vi "JKISM++ Example - Message API.vi"() -> ()   [LabVIEW 2014]
uses:
  user.lib/_NEVSTOP/JKI State Machine++/JKI State Machine++.lvlib
panel:
  out "Arguments 3":string
  out "Arguments 2":string
  out "Arguments":string
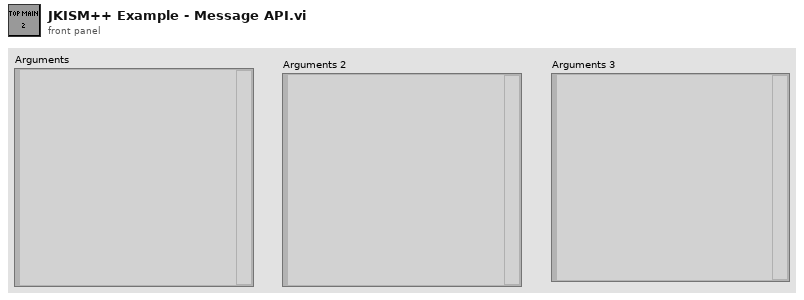
[diagram p1: front panel]
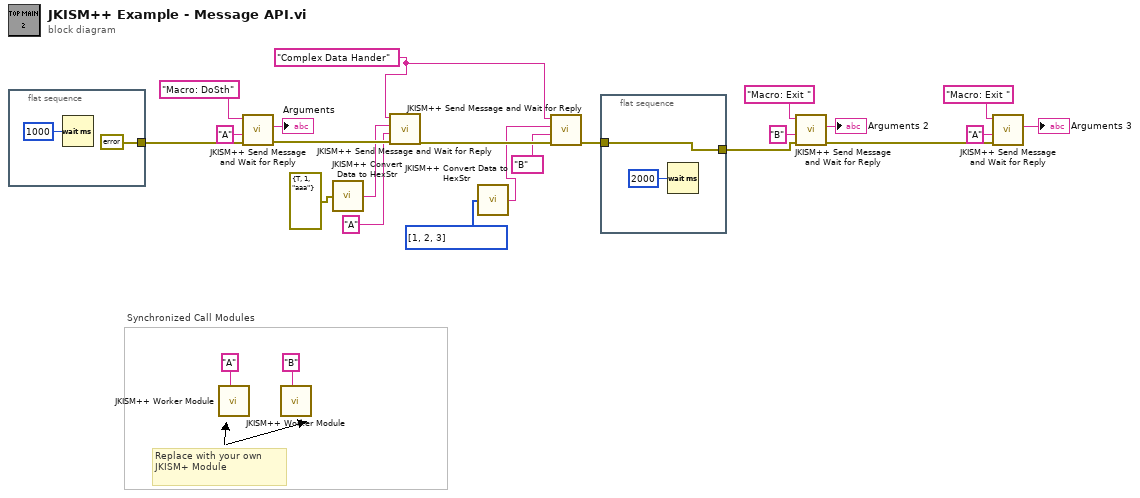
[diagram p0: block diagram]
diagram:
  w9 = "Complex Data Hander" ("State(s) in Front (\"\")")
  # "Synchronized Call Modules"
  # "Replace with your own JKISM+ Module"
  n1 = flat-sequence {
    tunnel: [errorcluster {"status"=FALSE, "code"=0, "source"=""} ("Error In (no error)")] -> w15
    frame #0 {
      n2 = Wait (ms)(milliseconds to wait=u32 1000) -> ()  [unwired: 1 out]
    }
  }
  n3 = call "JKISM++ Worker Module.vi"("Name(\"\" to use uuid)"="A" ("Name")) -> ()  [unwired: 11 in]
  n4 = call "JKISM++ Send Message and Wait for Reply.vi"("Error In (no error)"=w15, "Target Module"="A" ("Dest Module"), "State"="Macro: DoSth" ("State(s) in Front (\"\")")) -> ("error out"=w11:errorcluster, "Arguments"=→"Arguments":string)  [unwired: 7 in]
  n5 = call "JKISM++ Worker Module.vi"("Name(\"\" to use uuid)"="B" ("Name")) -> ()  [unwired: 11 in]
  n6 = call "JKISM++ Convert Data to HexStr.vi"("Variant"=errorcluster {"status"=TRUE, "code"=1, "source"="aaa"} ("Error In (no error)")) -> ("HEX String (0-9,A-F)"=w5:string)  [unwired: 8 in]
  n7 = call "JKISM++ Send Message and Wait for Reply.vi"("Error In (no error)"=w11, "Target Module"="A" ("Dest Module"), "Arguments (\"\")"=w5, "State"=w9) -> ("error out"=w10:errorcluster)  [unwired: 6 in, 1 out]
  n8 = call "JKISM++ Convert Data to HexStr.vi"("Variant"=i32[] [1, 2, 3]) -> ("HEX String (0-9,A-F)"=w4:string)  [unwired: 8 in]
  n9 = call "JKISM++ Send Message and Wait for Reply.vi"("Error In (no error)"=w10, "Target Module"="B" ("Dest Module"), "Arguments (\"\")"=w4, "State"=w9) -> ("error out"=w1:errorcluster)  [unwired: 6 in, 1 out]
  n10 = flat-sequence {
    tunnel: [w27] -> w2
    tunnel: w1 -> [w27]
    frame #0 {
      n11 = Wait (ms)(milliseconds to wait=u32 2000) -> ()  [unwired: 1 out]
    }
  }
  n12 = call "JKISM++ Send Message and Wait for Reply.vi"("Error In (no error)"=w2, "Target Module"="B" ("Dest Module"), "State"="Macro: Exit ") -> ("error out"=w16:errorcluster, "Arguments"=→"Arguments 2":string)  [unwired: 7 in]
  n13 = call "JKISM++ Send Message and Wait for Reply.vi"("Error In (no error)"=w16, "Target Module"="A" ("Dest Module"), "State"="Macro: Exit ") -> ("Arguments"=→"Arguments 3":string)  [unwired: 7 in, 1 out]
